vi "弧度至角度（单位）.vi"(1 "radian":dbl[unit]) -> (0 "degree":dbl[unit])   [LabVIEW 2012, in "几何工具.lvlib"]
doc: "功能：\n\n弧度转换为角度。\n\n输入：弧度。\n\n输出：角度，单位为度。\n\ncsxcs_366创建。"
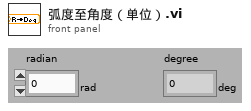
[diagram p1: front panel]
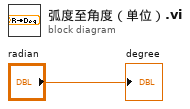
[diagram p0: block diagram]
diagram:
  "degree" <- "radian"
